vi "Create_CSV_From_JSON.vi"() -> ()   [LabVIEW 2020]
uses:
  <vilib>/Ngene/Deep Learning Toolkit/Toolkit/NN_Data/API/NN_Dims(C,H,W).ctl
  <vilib>/Ngene/Deep Learning Toolkit/Toolkit/Deep_Learning_Toolkit_by_Ngene.lvlib
  HyperParam_Investigation/Controls/Model_Info_and_Report.ctl
  HyperParam_Investigation/Controls/Feature_Layers_CFG.ctl
  <vilib>/Ngene/DeepLTK Anomaly Detection Addon/DeepLTK_Anomaly_Detection_Addon/API/Controls/MinMax.ctl
  <vilib>/Ngene/DeepLTK Anomaly Detection Addon/DeepLTK_Anomaly_Detection_Addon/DeepLTK_Anomaly_Detection_Addon.lvlib
  <vilib>/Ngene/DeepLTK Anomaly Detection Addon/DeepLTK_Anomaly_Detection_Addon/API/Controls/Eval_Results.ctl
panel:
  out "Progress":i32
  in  "error in":errorcluster
  out "error out":errorcluster
  in  "PatchCore Models Folder Path":path=path "D:/HyperParameter_Investigation/MVTec/bottle"
  in  "Results_Dest_Folder_Path":path=path "D:/HyperParameter_Investigation/MVTec/bottle"
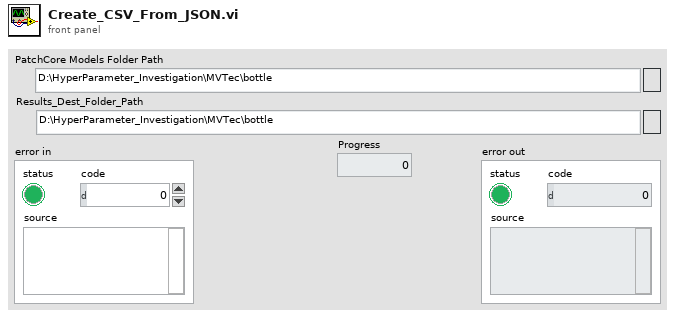
[diagram p1: front panel]
types:
  T1 = enum16{"open", "replace", "create", "open or create", "replace or create", "replace or create with confirmation"}
  T2 = typedef "Model_Info_and_Report.ctl" = cluster{"Name":string, "Feature Extractor":string, "Input3D_Custom_Dims":T3, "Coreset Size":i32, "J-L Proj. Dim.":i32, "Train_Time":dbl, "Inf_Time":dbl, "Feature_Layers":T4, "Eval Stats(Image)":T5, "Eval Stats(Pixel)":T5}
  T3 = typedef "Deep_Learning_Toolkit_by_Ngene.lvlib/NN_Dims(C,H,W).ctl" = cluster{"C":i32, "H":i32, "W":i32}
  T4 = typedef "Feature_Layers_CFG.ctl" = cluster{"Layer_ID":i32, "Patch_Size":i32}[]
  T5 = typedef "DeepLTK_Anomaly_Detection_Addon.lvlib/Eval_Results.ctl" = cluster{"Scores(Good)":T6, "Scores(Bad)":T6, "# of Samples(Good)":i32, "# of Samples(Bad)":i32, "AUROC":sgl, "F1_Max":sgl, "Thrshld(F1_Max)":sgl, "Prec.(F1_Max)":sgl, "Recall(F1_Max)":sgl, "FPR(F1_Max)":sgl, "FNR(F1_Max)":sgl}
  T6 = typedef "DeepLTK_Anomaly_Detection_Addon.lvlib/MinMax.ctl" = cluster{"Min":sgl, "Max":sgl}
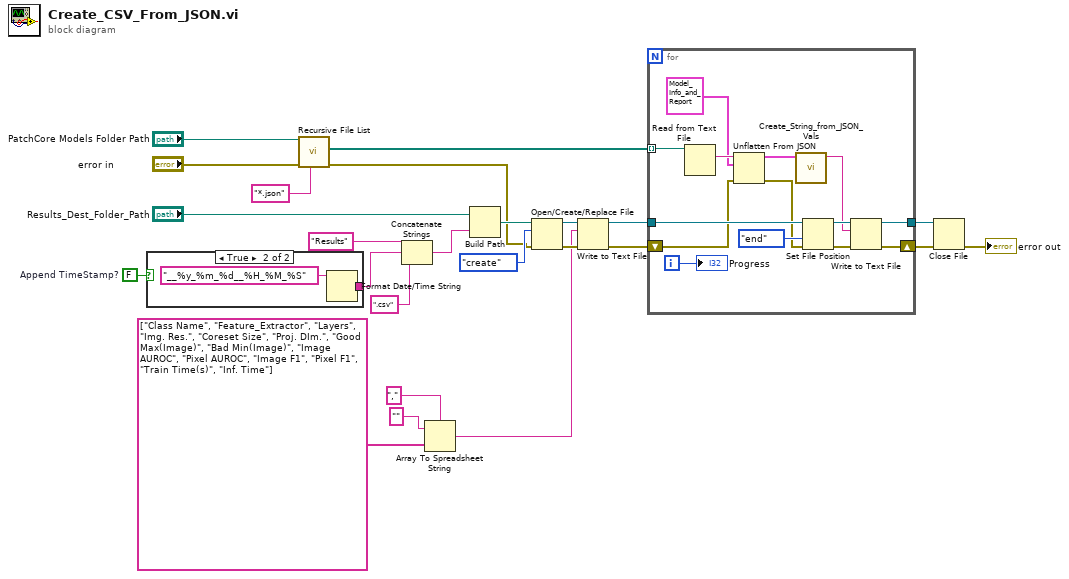
[diagram p0: block diagram]
diagram:
  w1 = FALSE  # Append TimeStamp?
  n1 = case shown="True" w1 {
    tunnel: [_ w26] -> w16
    frame False {
    }
    frame True {
      n2 = Format Date/Time String(time format string (%c)="__%y_%m_%d__%H_%M_%S") -> (date/time string=w26:string)  [unwired: 2 in]
    }
  }
  n3 = call <vilib>:"Recursive File List.vi"("pattern"="*.json", "error in (no error)"="error in", "Folder Path"="PatchCore Models Folder Path") -> ("error out"=w3:errorcluster, "All Files in Dir"=w10:path[])  [unwired: 4 in, 3 out]
  n4 = Concatenate Strings("Results" ("string"), w16, ".csv" ("string")) -> (w14:string)
  n5 = Array To Spreadsheet String(delimiter (Tab)=",", array=string[] ["Class Name", "Feature_Extractor", "Layers", "Img. Res.", "Coreset Size", "Proj. DIm.", "Good Max(Image)", "Bad Min(Image)", "Image AUROC", "Pixel AUROC", "Image F1", "Pixel F1", "Train Time(s)", "Inf. Time"] ("spreadsheet string"), 3:"" ("spreadsheet string")) -> (spreadsheet string=w7:string)
  n6 = Build Path(base path="Results_Dest_Folder_Path", name or relative path=w14) -> (appended path=w20:path)
  n7 = Open/Create/Replace File(file path (use dialog)=w20, error in=w3, operation (0:open)=T1."create") -> (refnum out=w19:refnum<file>, error out=w18:errorcluster)  [unwired: 3 in, 1 out]
  n8 = Write to Text File(file (use dialog)=w19, text=w7, error in=w18) -> (refnum out=w9:refnum<file>, error out=w8:errorcluster)  [unwired: 1 in, 1 out]
  n9 = for {
    tunnel: w10 -> [w40] mode=indexing
    tunnel: w9 -> [w33]
    tunnel: [w30] -> w6
    shift-right: [w29] -> w5
    shift-left: w8 -> [w32]
    i -> [w28]
    n10 = Read from Text File(file (use dialog)=w40) -> (text=w39:string)  [unwired: 3 in, 3 out]
    n11 = Unflatten From JSON(JSON string=w39, type and defaults=T2 {"Name"="", "Feature Extractor"="wrn_50_2_2_bnmerge", "Input3D_Custom_Dims"={"C"=0, "H"=0, "W"=-1}, "Coreset Size"=0, "J-L Proj. Dim."=0, "Train_Time"=0.0, "Inf_Time"=0.0, "Feature_Layers"=[{"Layer_ID"=8, "Patch_Size"=3}, {"Layer_ID"=16, "Patch_Size"=3}], "Eval Stats(Image)"={"Scores(Good)"={"Min"=0.0, "Max"=0.0}, "Scores(Bad)"={"Min"=0.0, "Max"=0.0}, "# of Samples(Good)"=0, "# of Samples(Bad)"=0, "AUROC"=0.0, "F1_Max"=0.0, "Thrshld(F1_Max)"=0.0, "Prec.(F1_Max)"=0.0, "Recall(F1_Max)"=0.0, "FPR(F1_Max)"=0.0, "FNR(F1_Max)"=0.0}, "Eval Stats(Pixel)"={"Scores(Good)"={"Min"=0.0, "Max"=0.0}, "Scores(Bad)"={"Min"=0.0, "Max"=0.0}, "# of Samples(Good)"=0, "# of Samples(Bad)"=0, "AUROC"=0.0, "F1_Max"=0.0, "Thrshld(F1_Max)"=0.0, "Prec.(F1_Max)"=0.0, "Recall(F1_Max)"=0.0, "FPR(F1_Max)"=0.0, "FNR(F1_Max)"=0.0}} ("Model_Info_and_Report"), error in (no error)=w32) -> (value=w38:T2, error out=w31:errorcluster)  [unwired: 4 in]
    n12 = call "Create_String_from_JSON_Vals.vi"("Model_Info_and_Report"=w38) -> ("String"=w34:string)  [unwired: 10 in]
    n13 = Set File Position(refnum=w33, from (0:start)=enum16{"start", "end", "current"}."end", error in=w31) -> (refnum out=w37:refnum<file>, error out=w36:errorcluster)  [unwired: 1 in]
    n14 = Write to Text File(file (use dialog)=w37, text=w34, error in=w36) -> (refnum out=w30:refnum<file>, error out=w29:errorcluster)  [unwired: 1 in, 1 out]
    "Progress" <- w28
  }
  n15 = Close File(refnum=w6, error in=w5) -> (error out=→"error out":errorcluster)  [unwired: 1 out]
